vi "Create PPL.vi"(0 "configuration":T1, 11 "error in":errorcluster) -> (4 "project refnum":refnum<vi>, 15 "error out":errorcluster)   [LabVIEW 2021, in "InstrumentStudio Plug-In Editor.lvlib"]
uses:
  InstrumentStudio Plug-In Editor.lvlib
  Data Holder.ctl
  <vilib>/AppBuilder/AB_API/PPL/NI_AB_API_PPL.lvclass
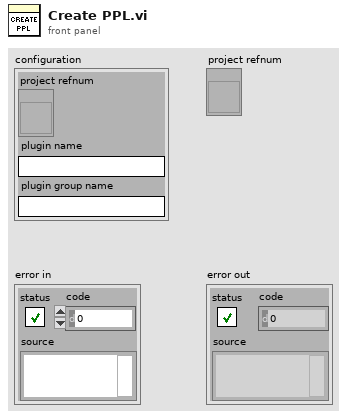
[diagram p1: front panel]
types:
  T1 = typedef "InstrumentStudio Plug-In Editor.lvlib/Data Holder.ctl" = cluster{"project refnum":refnum<vi>, "plugin name":string, "plugin group name":string}
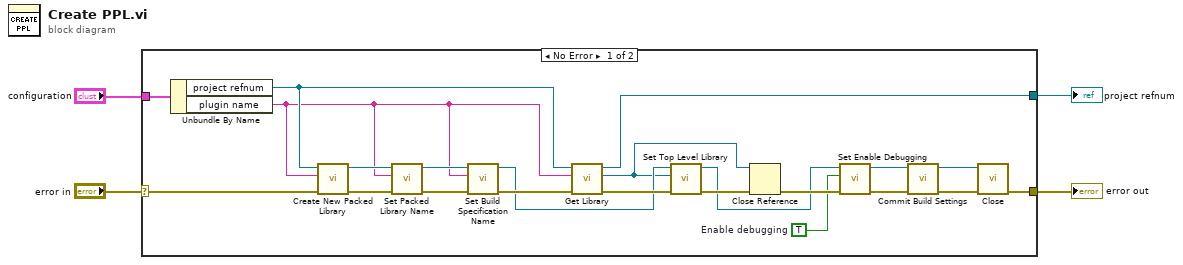
[diagram p0: block diagram]
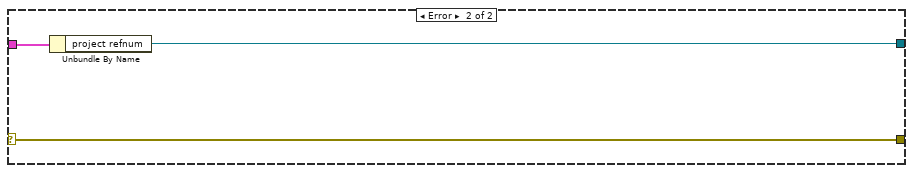
[diagram p2: hidden frame]
diagram:
  n1 = case shown="No Error" "error in" {
    selector: "error in" -> [w17 w29]
    tunnel: [w22 w29] -> w3
    tunnel: [w10 w28] -> w2
    tunnel: "configuration" -> [w6 w27]
    frame No Error {
      w5 = TRUE  # Enable debugging
      n2 = Unbundle By Name(w6) -> ("project refnum"=w9:refnum<vi>, "plugin name"=w8:string)
      n3 = call <vilib>:"Create New Packed Library.vi"("error in (no error)"=w17, "Build specification name"=w8, "Project Refnum"=w9) -> ("error out"=w21:errorcluster, "PPL out"=w20:refnum<class "NI_AB_API_PPL.lvclass">)  [unwired: 7 in]
      n4 = call-dynamic "Set Packed Library Name.vi"("error in (no error)"=w21, "Packed library name"=w8, "PPL in"=w20) -> ("error out"=w23:errorcluster, "PPL out"=w24:refnum<class "NI_AB_API_PPL.lvclass">)  [unwired: 7 in]
      n5 = call-dynamic "Set Build Specification Name.vi"("error in (no error)"=w23, "Build Specification Name"=w8, "NI_AB_API_PPL in"=w24) -> ("error out"=w16:errorcluster, "NI_AB_API_PPL out"=w12:refnum<class "NI_AB_API_PPL.lvclass">)  [unwired: 7 in]
      n6 = call "Get Library.vi"("error in"=w16, "library name"=w8, "project refnum in"=w9) -> ("error out"=w15:errorcluster, "library refnum"=w7:refnum<vi>, "project refnum out"=w10:refnum<vi>)  [unwired: 5 in, 1 out]
      n7 = call-dynamic "Set Top Level Library.vi"("error in (no error)"=w15, "ProjectItem Refnum"=w7, "PPL in"=w12) -> ("error out"=w14:errorcluster, "PPL out"=w11:refnum<class "NI_AB_API_PPL.lvclass">)  [unwired: 7 in]
      n8 = Close Reference(reference=w7, error in (no error)=w14) -> (error out=w13:errorcluster)
      n9 = call-dynamic "Set Enable Debugging.vi"("error in (no error)"=w13, "Enable debugging (false)"=w5, "PPL in"=w11) -> ("error out"=w19:errorcluster, "PPL out"=w18:refnum<class "NI_AB_API_PPL.lvclass">)  [unwired: 7 in]
      n10 = call-dynamic "Commit Build Settings.vi"("error in (no error)"=w19, "PPL in"=w18) -> ("error out"=w26:errorcluster, "PPL out"=w25:refnum<class "NI_AB_API_PPL.lvclass">)  [unwired: 8 in]
      n11 = call-dynamic "Close.vi"("error in (no error)"=w26, "DLL in"=w25) -> ("error out"=w22:errorcluster)  [unwired: 9 in]
    }
    frame Error {
      n12 = Unbundle By Name(w27) -> ("project refnum"=w28:refnum<vi>)
    }
  }
  "error out" <- w3
  "project refnum" <- w2
